vi "Pop Up.vi"(11 "Dev Actor in":refnum<class "Dev Actor.lvclass">) -> (3 "Dev Actor out":refnum<class "Dev Actor.lvclass">)   [LabVIEW 2021, in "Dev Actor.lvlib" / "Dev Actor.lvclass"]
uses:
  Dev Actor.lvclass
  C:/Program Files/National Instruments/LabVIEW 2021/vi.lib/jettl/jettl/Actor/Actor/Actor.lvclass
  Dev Actor.lvclass/Dev Actor.ctl
  <vilib>/jettl/jettl/Actor/Msgs/Create/Create Msg/Create Msg.lvclass
  C:/Program Files/National Instruments/LabVIEW 2021/vi.lib/jettl/jettl/Actor/Msg/Msg.lvclass
  <vilib>/jettl/jettl/Actor/Msgs/Destroy/Destroy Msg/Destroy Msg.lvclass
  <vilib>/jettl/jettl/Actor/Actor/Actor.lvclass
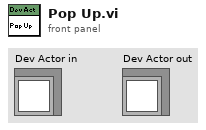
[diagram p1: front panel]
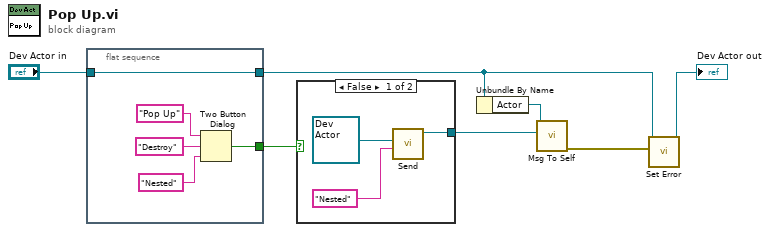
[diagram p0: block diagram]
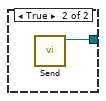
[diagram p2: hidden frame]
diagram:
  n1 = flat-sequence {
    tunnel: [w12] -> w3
    tunnel: "Dev Actor in" -> [w12]
    tunnel: [w9] -> w4
    frame #0 {
      n2 = Two Button Dialog(message="Pop Up", 1:"Nested" ("F button name (\"Cancel\")"), 2:"Destroy" ("T button name (\"OK\")")) -> (T button?=w9:bool)
    }
  }
  n3 = case shown="False" w4 {
    tunnel: [w15 w16] -> w5
    frame False {
      n4 = call <vilib>:"Send.vi"("Alias"="Nested" ("Nested Alias"), "Actor"=refnum<class "Dev Actor.lvclass"> refnum ("Dev Actor.lvlib:Dev Actor.lvclass")) -> ("Create Msg out"=w15:refnum<class "Create Msg.lvclass">)  [unwired: 9 in]
    }
    frame True {
      n5 = call <vilib>:"Send.vi"() -> ("Destroy Msg out"=w16:refnum<class "Destroy Msg.lvclass">)  [unwired: 11 in]
    }
  }
  n6 = Unbundle By Name(w3) -> ("Actor"=w6:refnum<class "Actor.lvclass">)
  n7 = call-dynamic "Msg To Self.vi"("Msg"=w5, "Actor in"=w6) -> ("error out"=w1:errorcluster)  [unwired: 9 in]
  n8 = call-dynamic "Set Error.vi"("Merge"=w1, "Dev Actor in"=w3) -> ("Dev Actor out"=→"Dev Actor out":refnum<class "Dev Actor.lvclass">)  [unwired: 9 in]
